vi "CAN GIP Test.vi"(8 "error in":errorcluster, 10 "Interface":refnum<k21>="CAN4", 11 "SequenceContext":refnum<k7>) -> (0 "error out":errorcluster={"status"=TRUE, "code"=-1074384711, "source"="XNET Create Session (Signal Input Single-point).vi:6590002<APPEND>\n\n<b>Complete call chain:</b>\r\n     XNET Create Session (Signal Input Single-point).vi:6590002\r\n     CAN GIP.lvlib:GIP CAN Wrapper.vi:2150001\r\n     CAN GIP.lvlib:CAN GIP Test.vi"}, 3 "output":dbl[](array[numeric]))   [LabVIEW 2021, in "CAN GIP.lvlib"]
uses:
  CAN GIP.lvlib
  Private Controls/CAN States.ctl
  Private Controls/Setting.ctl
  2366c070-ee15-47bc-b72b-1957ca1c4b1d.vi
  <vilib>/addons/TestStand/_TSUtility.llb/TestStand - Get Property Value (String).vi
  <vilib>/addons/TestStand/_TSUtility.llb/TestStand - Get Property Value (Number).vi
  <vilib>/addons/TestStand/_TSUtility.llb/TestStand - Get Property Value (Boolean).vi
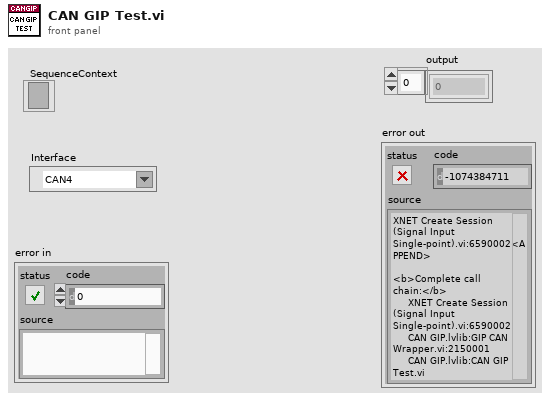
[diagram p1: front panel]
types:
  T1 = typedef "CAN GIP.lvlib/Setting.ctl" = cluster{"Termination":u32, "Baud Rate":u64, "Interface":refnum<k21>, "XNET Database":refnum<k21>, "ECU":refnum<k21>}
  T2 = typedef "CAN GIP.lvlib/CAN States.ctl" = enum16{"Init", "Config", "Read Signals", "Write Signals", "Close"}
  T3 = typedef "TestStand - Status Monitor.ctl" = cluster{"Sequence Context":refnum<k7>, "Execution":refnum<k7>, "Termination Monitor":refnum<k7>}
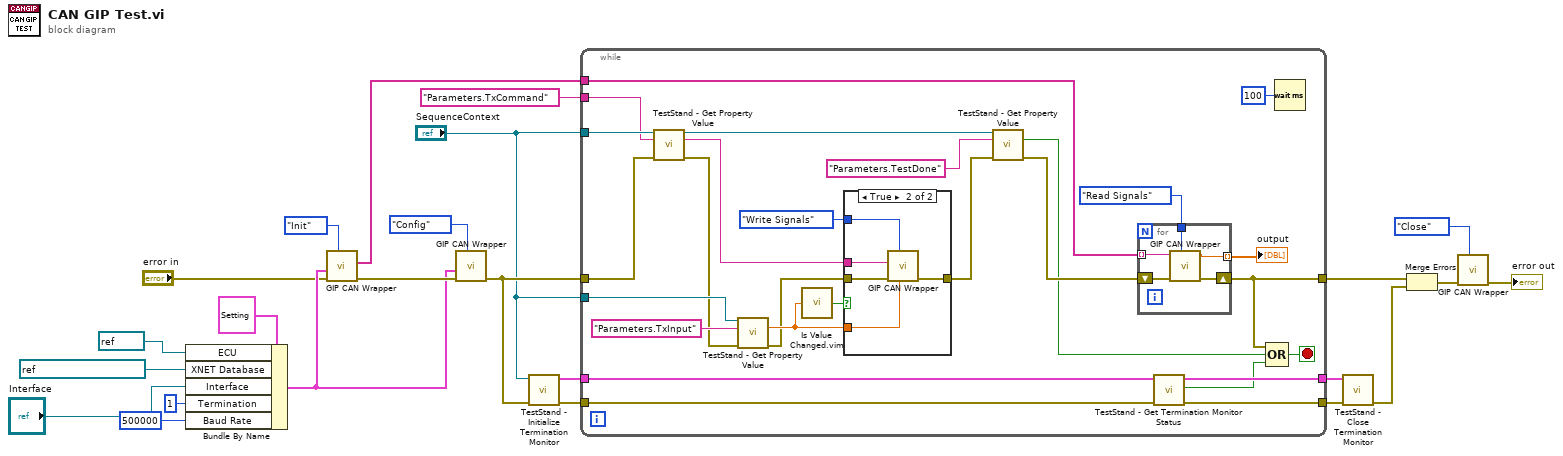
[diagram p0: block diagram]
diagram:
  n1 = Bundle By Name(cluster=T1 {"Termination"=1, "Baud Rate"=125000, "Interface"="CAN1", "XNET Database"="GIP_CAN_Database", "ECU"="GIP\nGIP_CAN_Database"} ("Setting"), "ECU"=refnum<k21> "GIP\ncan_messages_818", "XNET Database"=refnum<k21> "can_messages_818", "Interface"="Interface", "Termination"=u32 1, "Baud Rate"=u64 500000) -> (w18:T1)
  n2 = call "GIP CAN Wrapper.vi"("States"=CAN_States."Init" ("CAN States"), "error in"="error in", "Setting"=w18) -> ("error out"=w23:errorcluster, "Rx SigNames"=w3:string[])  [unwired: 6 in, 1 out]
  n3 = call "GIP CAN Wrapper.vi"("States"=CAN_States."Config" ("CAN States"), "error in"=w23, "Setting"=w18) -> ("error out"=w17:errorcluster)  [unwired: 6 in, 2 out]
  n4 = call <vilib>:"TestStand - Initialize Termination Monitor.vi"("error in (no error)"=w17, "Sequence Context In"="SequenceContext") -> ("error out"=w16:errorcluster, "Status Monitor Out"=w14:T3)  [unwired: 8 in]
  n5 = while {
    tunnel: [w42] -> w11
    tunnel: w17 -> [w35]
    tunnel: w3 -> [w48]
    tunnel: w16 -> [w47]
    tunnel: [w43] -> w15
    tunnel: w14 -> [w46]
    tunnel: [w45] -> w13
    tunnel: "SequenceContext" -> [w34]
    tunnel: "Parameters.TxCommand" ("Lookup String") -> [w32]
    tunnel: "SequenceContext" -> [w29]
    stop <- w44 stop-if-true
    n6 = call-poly <vilib>:"TestStand - Get Property Value.vi"("Sequence Context In"=w34, "Lookup String"=w32, "error in (no error)"=w35) -> ("Sequence Context Out"=w33:refnum<k7>, "Value"=w31:string, "error out"=w26:errorcluster)  [unwired: 10 in]
    n7 = call-poly <vilib>:"TestStand - Get Property Value.vi"("Sequence Context In"=w29, "Lookup String"="Parameters.TxInput", "error in (no error)"=w26) -> ("Value"=w28:dbl, "error out"=w25:errorcluster)  [unwired: 10 in, 1 out]
    n8 = call "Is Value Changed.vim"("value"=w28) -> ("changed or first call?"=w27:bool)
    n9 = case shown="True" w27 {
      tunnel: w25 -> [w52 w57]
      tunnel: [w52 w56] -> w39
      tunnel: CAN_States."Write Signals" ("CAN States") -> [_ w55]
      tunnel: w28 -> [_ w54]
      tunnel: w31 -> [_ w53]
      frame False {
      }
      frame True {
        n10 = call "GIP CAN Wrapper.vi"("Signal Write"=w54, "States"=w55, "error in"=w57, "Tx Signal In"=w53) -> ("error out"=w56:errorcluster)  [unwired: 5 in, 2 out]
      }
    }
    n11 = call-poly <vilib>:"TestStand - Get Property Value.vi"("Sequence Context In"=w33, "Lookup String"="Parameters.TestDone", "error in (no error)"=w39) -> ("Value"=w36:bool, "error out"=w38:errorcluster)  [unwired: 10 in, 1 out]
    n12 = for {
      tunnel: CAN_States."Read Signals" ("CAN States") -> [w62]
      tunnel: w48 -> [w60] mode=indexing
      shift-right: [w59] -> w42
      shift-left: w38 -> [w61]
      tunnel: [w58] -> w40 mode=indexing
      n13 = call "GIP CAN Wrapper.vi"("States"=w62, "error in"=w61, "Rx Signal In"=w60) -> ("error out"=w59:errorcluster, "Signal out"=w58:dbl)  [unwired: 6 in, 1 out]
    }
    "output" <- w40
    n14 = call <vilib>:"TestStand - Get Termination Monitor Status.vi"("error in (no error)"=w47, "Status Monitor In"=w46) -> ("error out"=w43:errorcluster, "Terminating or Aborting"=w41:bool, "Status Monitor Out"=w45:T3)  [unwired: 7 in]
    n15 = Compound Arithmetic op=OR(w42, w36, w41) -> (w44:bool)
    n16 = Wait (ms)(milliseconds to wait=u32 100) -> ()  [unwired: 1 out]
  }
  n17 = call <vilib>:"TestStand - Close Termination Monitor.vi"("error in (no error)"=w15, "Status Monitor In"=w13) -> ("error out"=w12:errorcluster)  [unwired: 9 in]
  n18 = Merge Errors(w11, w12) -> (w10:errorcluster)
  n19 = call "GIP CAN Wrapper.vi"("States"=CAN_States."Close" ("CAN States"), "error in"=w10) -> ("error out"=→"error out":errorcluster)  [unwired: 7 in, 2 out]
